vi "Init Data.vi"(8 "error in (no error)":errorcluster, 10 "Data Object":refnum<class "Factory Plugin Framework.lvclass">, 11 "Skyworks Spur Test in":refnum<class "Skyworks Spur Test.lvclass">) -> (0 "error out":errorcluster, 3 "Skyworks Spur Test out":refnum<class "Skyworks Spur Test.lvclass">)   [LabVIEW 2018, in "Skyworks Spur Test.lvlib" / "Skyworks Spur Test.lvclass"]
uses:
  Skyworks Spur Test.lvclass
  Plugins/FPF.lvlibp/Factory Plugin Framework.lvclass
  Plugins/Measurement Interface.lvlibp/Measurement Interface.lvclass
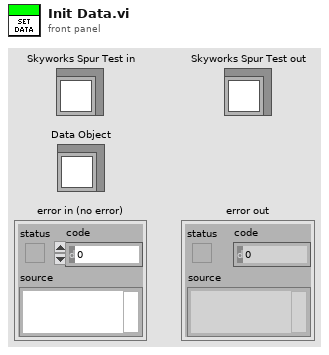
[diagram p1: front panel]
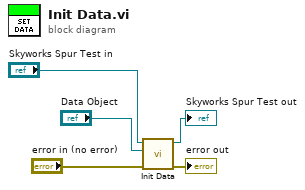
[diagram p0: block diagram]
diagram:
  n1 = call-parent "Init Data.vi"("error in (no error)"="error in (no error)", "Data Object"="Data Object", "Measurement Interface in"="Skyworks Spur Test in") -> ("error out"=→"error out":errorcluster, "Measurement Interface out"=→"Skyworks Spur Test out":refnum<class "Skyworks Spur Test.lvclass">)  [unwired: 7 in]
